vi "VG_DCIR+OUIouNON.vi"() -> ()   [LabVIEW 2020]
panel:
  out "VG_DCIR+ ?":bool
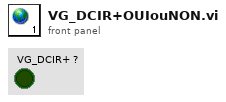
[diagram p1: front panel]
diagram:
